vi "Start BLE Server.vi"(8 "Error In":errorcluster) -> (0 "Error Out":errorcluster)   [LabVIEW 2016]
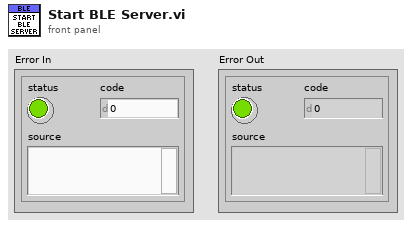
[diagram p1: front panel]
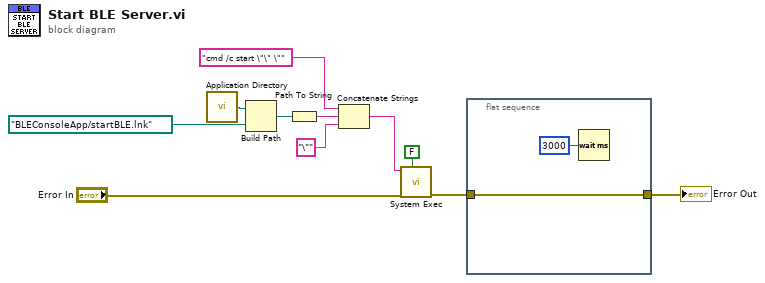
[diagram p0: block diagram]
diagram:
  n1 = call <vilib>:"Application Directory.vi"() -> ("Application Directory"=w11:path)
  n2 = Build Path(base path=w11, name or relative path=path "BLEConsoleApp/startBLE.lnk") -> (appended path=w9:path)
  n3 = Path To String(path=w9) -> (string=w7:string)
  n4 = Concatenate Strings("cmd /c start \"\" \"" ("string"), w7, "\"" ("string")) -> (w6:string)
  n5 = call <vilib>:"System Exec.vi"("wait until completion? (T)"=FALSE, "error in (no error)"="Error In", "command line"=w6) -> ("error out"=w2:errorcluster)  [unwired: 5 in, 3 out]
  n6 = flat-sequence {
    tunnel: w2 -> [w13]
    tunnel: [w13] -> w1
    frame #0 {
      n7 = Wait (ms)(milliseconds to wait=u32 3000) -> ()  [unwired: 1 out]
    }
  }
  "Error Out" <- w1
